vi "Occupancy Grid Drawing.vi"(1 "Particle Points":dbl[][](array[numeric])) -> (0 "Output Occupancy Grid":dbl[][](array[numeric]))   [LabVIEW 2014]
panel:
  out "Occupancy Grid Drawing":dbl[][](graph)
  out "Intermediate Value Array":dbl[][](array[numeric])
  # "CM(X), CM(Y), Left X, Right X"
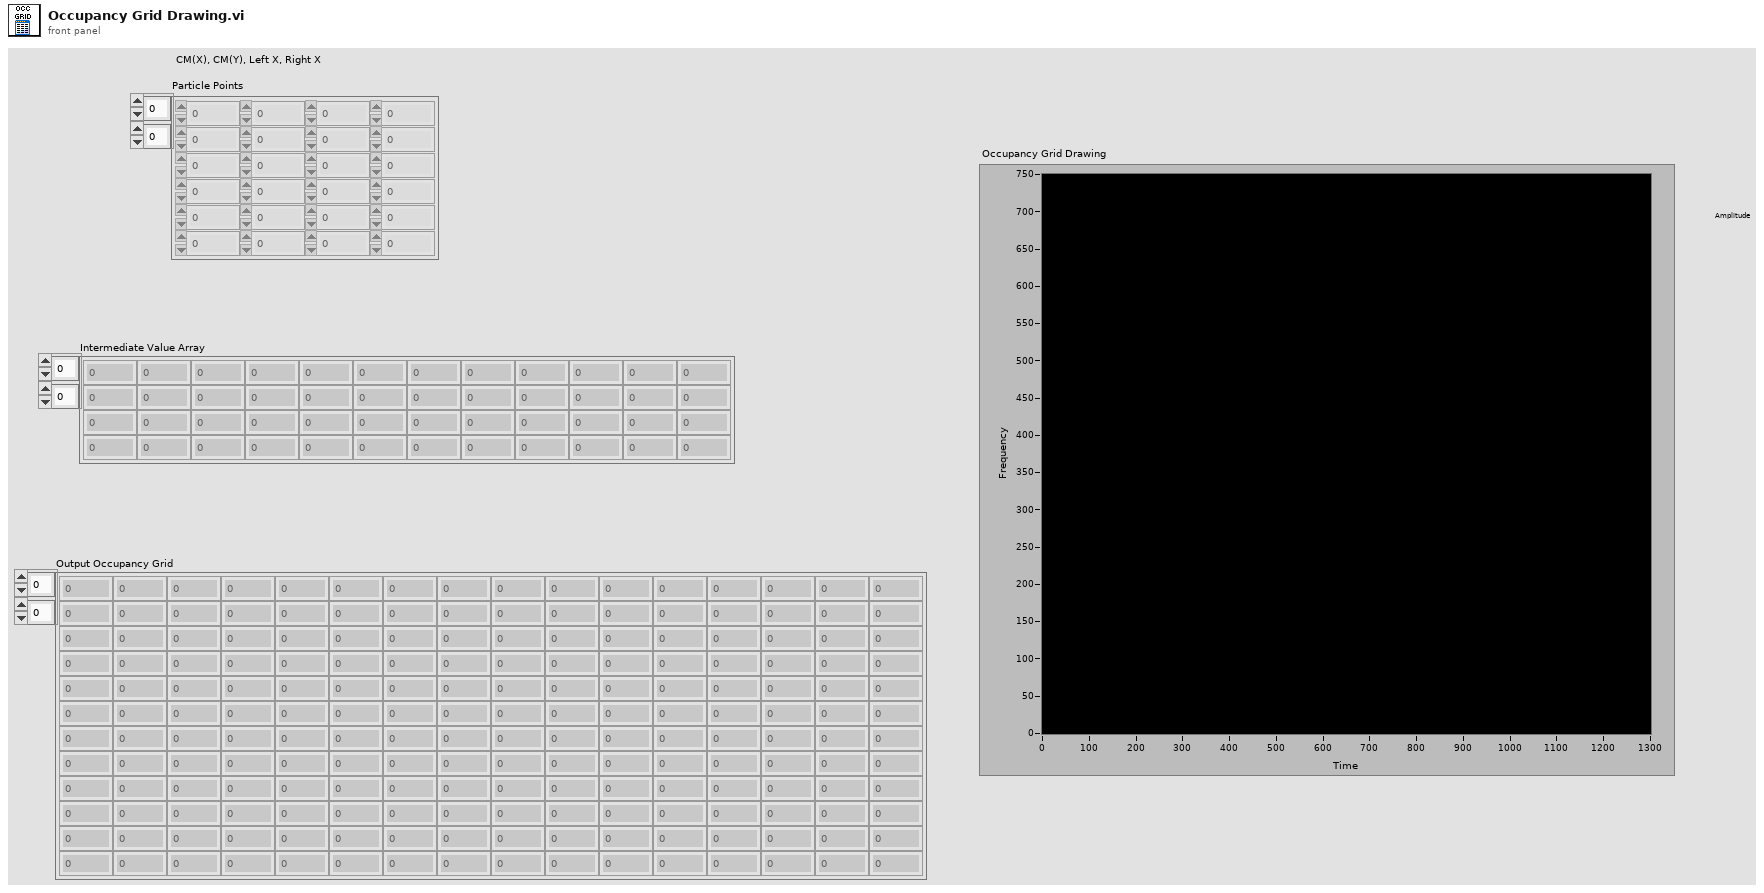
[diagram p1: front panel]
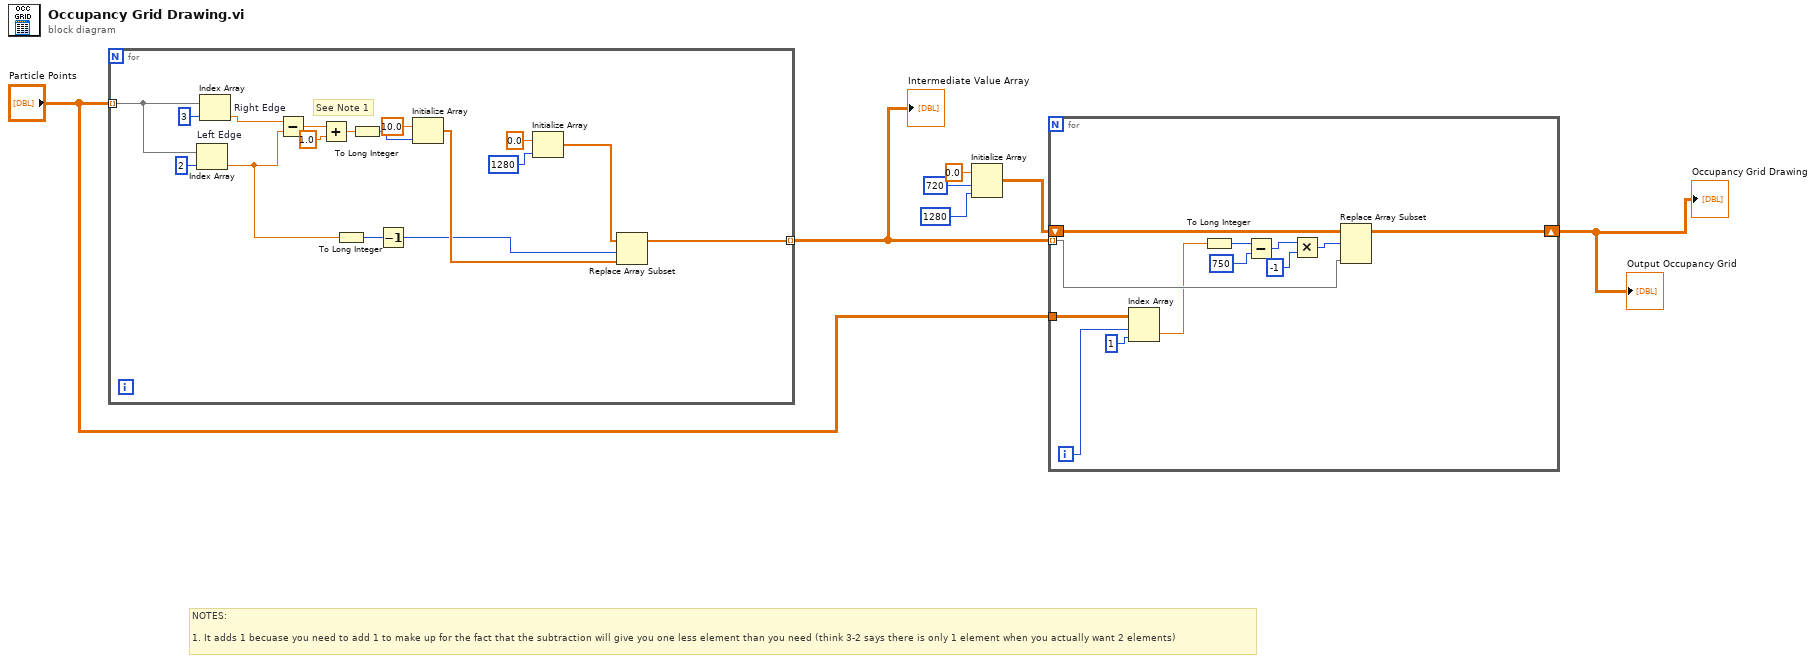
[diagram p0: block diagram]
diagram:
  # "NOTES:\n\n1. It adds 1 becuase you need to add 1 to make up for the fact that the subtraction will give you one less element than you need (think 3-2 says there is only 1 element when you actually want 2 elements)"
  n1 = for {
    tunnel: "Particle Points" -> [w21] mode=indexing
    tunnel: [w11] -> w4 mode=indexing
    # "See Note 1"
    n2 = Index Array "Left Edge"(array=w21, index=2) -> (element=w10:dbl)
    n3 = Index Array "Right Edge"(array=w21, index=3) -> (element=w12:dbl)
    n4 = Subtract(x=w12, y=w10) -> (x-y=w20:dbl)
    n5 = Add(x=w20, y=1.0) -> (x+y=w18:dbl)
    n6 = To Long Integer(number=w10) -> (32bit integer=w9:i32)
    n7 = To Long Integer(number=w18) -> (32bit integer=w16:i32)
    n8 = Decrement(x=w9) -> (x-1=w8:i32)
    n9 = Initialize Array(10.0 ("element"), w16) -> (w14:dbl[])
    n10 = Initialize Array(0.0 ("element"), 1280 ("dimension size")) -> (w13:dbl[])
    n11 = Replace Array Subset(array=w13, new element=w14, index=w8) -> (w11:dbl[])
  }
  "Intermediate Value Array" <- w4
  n12 = Initialize Array(0.0 ("element"), 720 ("dimension size"), 1280 ("dimension size")) -> (w2:dbl[][])
  n13 = for {
    tunnel: w4 -> [w33] mode=indexing
    tunnel: "Particle Points" -> [w36]
    shift-right: [w31] -> w1
    shift-left: w2 -> [w34]
    i -> [w30]
    n14 = Index Array(array=w36, index (row)=w30, index (col)=1 ("disabled index (col)")) -> (element=w32:dbl)
    n15 = To Long Integer(number=w32) -> (32bit integer=w29:i32)
    n16 = Subtract(x=w29, y=750) -> (x-y=w27:i32)
    n17 = Multiply(x=w27, y=-1) -> (x*y=w25:i32)
    n18 = Replace Array Subset(array=w34, new element=w33, index (row)=w25) -> (w31:dbl[][])  [unwired: 1 in]
  }
  "Output Occupancy Grid" <- w1
  "Occupancy Grid Drawing" <- w1
